vi "Format LogRecord.vi"(8 "error in":errorcluster, 10 "LogRecord":refnum<class "LogRecord.lvclass">, 11 "JSONLFormatter in":refnum<class "JSONLFormatter.lvclass">) -> (0 "error out":errorcluster, 2 "LogLine":string)   [LabVIEW 2024, in "hse-logger.lvlib" / "JSONLFormatter.lvclass"]
doc: "Format the Log Record.\n\n____\nHAMPEL SOFTWARE ENGINEERING v2.2.2 (2025-01-16 15:41)"
uses:
  <vilib>/Hampel Software Engineering/HSE Logger/Formatter/JSONLFormatter/JSONLFormatter.lvclass
  C:/Program Files (x86)/National Instruments/LabVIEW 2024/vi.lib/Hampel Software Engineering/HSE Logger/Formatter/Formatter.lvclass
  <vilib>/Hampel Software Engineering/HSE Logger/LogRecord/LogRecord.lvclass
  <vilib>/Hampel Software Engineering/HSE Logger/LogRecord/LogRecord.lvclass/LogRecord.ctl
  <vilib>/Hampel Software Engineering/HSE Logger/Formatter/Formatter.lvclass/Formatter.ctl
  <vilib>/Hampel Software Engineering/HSE Logger/Formatter/JSONLFormatter/JSONLFormatter.lvclass/JSONLFormatter.ctl
  <vilib>/Hampel Software Engineering/HSE Logger/Formatter/Formatter.lvclass
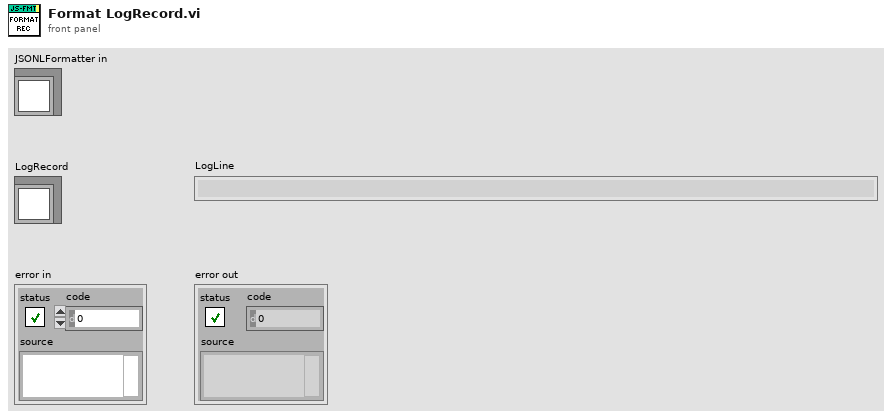
[diagram p1: front panel]
types:
  T1 = typedef "hse-logger.lvlib/LogLevel.ctl" = enum16{"DEBUG", "INFO", "WARNING", "ERROR", "CRITICAL"}
  T2 = typedef "hse-logger.lvlib/JSONLFormatter.lvclass/Format--cluster.ctl" = cluster{"time":string, "log_level":string, "message":string, "call_chain":string, "error_code":string, "source":string}
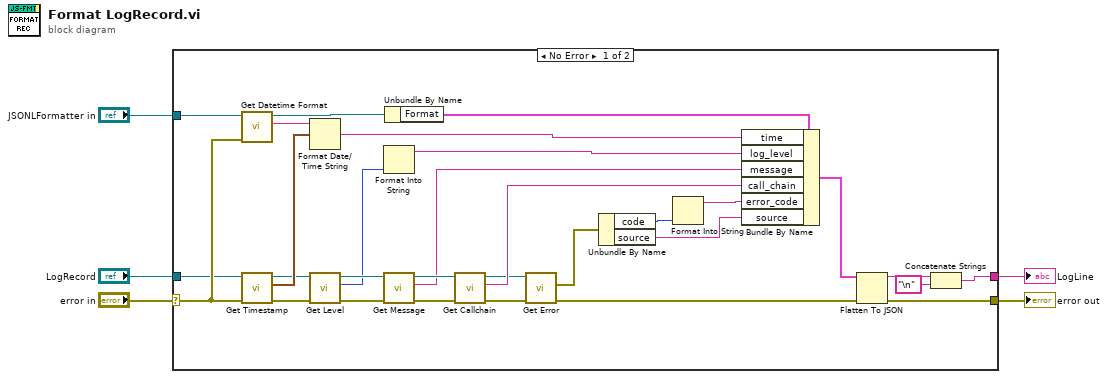
[diagram p0: block diagram]
diagram:
  n1 = case shown="No Error" "error in" {
    selector: "error in" -> [w34 w36]
    tunnel: [w35 w36] -> w5
    tunnel: [w25 _] -> w3
    tunnel: "LogRecord" -> [w23 _]
    tunnel: "JSONLFormatter in" -> [w27 _]
    frame No Error {
      n2 = call <vilib>:"Get Datetime Format.vi"("error in"=w34, "Formatter in"=w27) -> ("Datetime Format"=w26:string, "Formatter out"=w24:refnum<class "JSONLFormatter.lvclass">)  [unwired: 7 in, 1 out]
      n3 = call <vilib>:"Get Timestamp.vi"("error in"=w34, "LogRecord in"=w23) -> ("error out"=w33:errorcluster, "Created"=w19:timestamp, "LogRecord out"=w12:refnum<class "LogRecord.lvclass">)  [unwired: 7 in]
      n4 = Format Date/Time String(time format string (%c)=w26, seconds (now)=w19) -> (date/time string=w18:string)  [unwired: 1 in]
      n5 = call <vilib>:"Get Level.vi"("error in"=w33, "LogRecord in"=w12) -> ("error out"=w32:errorcluster, "Level"=w7:T1, "LogRecord out"=w21:refnum<class "LogRecord.lvclass">)  [unwired: 7 in]
      n6 = Format Into String(w7) -> (resulting string=w14:string)  [unwired: 3 in, 1 out]
      n7 = call <vilib>:"Get Message.vi"("error in"=w32, "LogRecord in"=w21) -> ("error out"=w31:errorcluster, "Message"=w17:string, "LogRecord out"=w20:refnum<class "LogRecord.lvclass">)  [unwired: 7 in]
      n8 = Unbundle By Name(w24) -> ("Format"=w11:T2)
      n9 = call <vilib>:"Get Callchain.vi"("error in"=w31, "LogRecord in"=w20) -> ("error out"=w30:errorcluster, "Callchain"=w16:string, "LogRecord out"=w6:refnum<class "LogRecord.lvclass">)  [unwired: 7 in]
      n10 = call <vilib>:"Get Error.vi"("error in"=w30, "LogRecord in"=w6) -> ("error out"=w29:errorcluster, "Error"=w28:errorcluster)  [unwired: 7 in, 1 out]
      n11 = Unbundle By Name(w28) -> ("code"=w9:i32, "source"=w10:string)
      n12 = Format Into String(w9) -> (resulting string=w8:string)  [unwired: 3 in, 1 out]
      n13 = Bundle By Name(cluster=w11, "time"=w18, "log_level"=w14, "message"=w17, "call_chain"=w16, "error_code"=w8, "source"=w10) -> (w15:T2)
      n14 = Flatten To JSON(anything=w15, error in (no error)=w29) -> (JSON string=w22:string, 11:w35:errorcluster)  [unwired: 1 in]
      n15 = Concatenate Strings(w22, "\n" ("string")) -> (w25:string)
    }
    frame Error {
    }
  }
  "error out" <- w5
  "LogLine" <- w3
